vi "USB Write User Data.vi"(7 "DataLen":i32, 9 "pWriteData":u8[](array[numeric])=array[20480 elements], 10 "OffsetAddr":i32, 11 "DevIndex":i32) -> (3 "function return":bool)   [LabVIEW 2010, in "usb_device.lvlib"]
doc: "bool WINAPI USB_WriteUserData(int DevIndex,int OffsetAddr,unsigned char *pWriteData,int DataLen);"
uses:
  usb_device.lvlib
  USB2XXX.dll
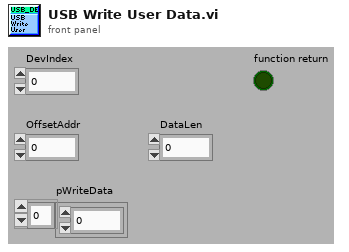
[diagram p1: front panel]
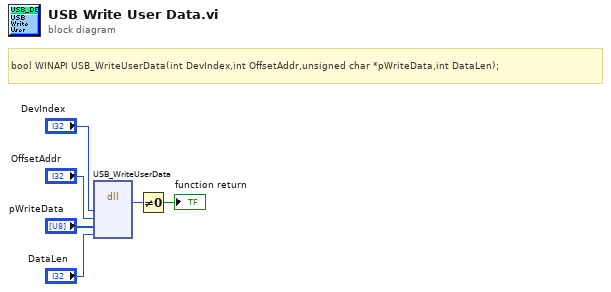
[diagram p0: block diagram]
diagram:
  # "bool WINAPI USB_WriteUserData(int DevIndex,int OffsetAddr,unsigned char *pWriteData,int DataLen);"
  n1 = dll-call lib="G:/OtherWork/USB2XXX_Example/trunk/Labview/PublicFiles/usb_device/USB2XXX.*" fn="USB_WriteUserData"("DevIndex"="DevIndex", "OffsetAddr"="OffsetAddr", "pWriteData"="pWriteData", "DataLen"="DataLen") -> (w5:u8)  [unwired: 7 in, 2 out]
  n2 = Not Equal To 0?(x=w5) -> (x != 0?=→"function return":bool)
